vi "Roller IR Logic.vi"(11 "Roller Command In":T2) -> (3 "Roller Command Out":T2, 5 "State":T1)   [LabVIEW 2013]
uses:
  Roller Control.ctl
  Roller Mode.ctl
  Common Code/IR Logic State.ctl
  Common Code/Change Detect Boolean.vi
  Utilities/TimeManager.vi
  Robot Global Data.vi
panel:
  out "IR":cluster{"f":dbl, "f":dbl, "f":dbl}(graph)
  out "Chart":cluster{dbl}(graph)
  in  "Roller/Back IR":bool caption="Back"
  in  "Roller/Center IR":bool caption="Center"
  in  "Roller/Front IR":bool caption="Front"
  in  "To Center Timeout":dbl
  in  "Entry Timeout":dbl
  in  "Verify Center time":dbl
  # "Debugging controls under this box"
  # "IR"
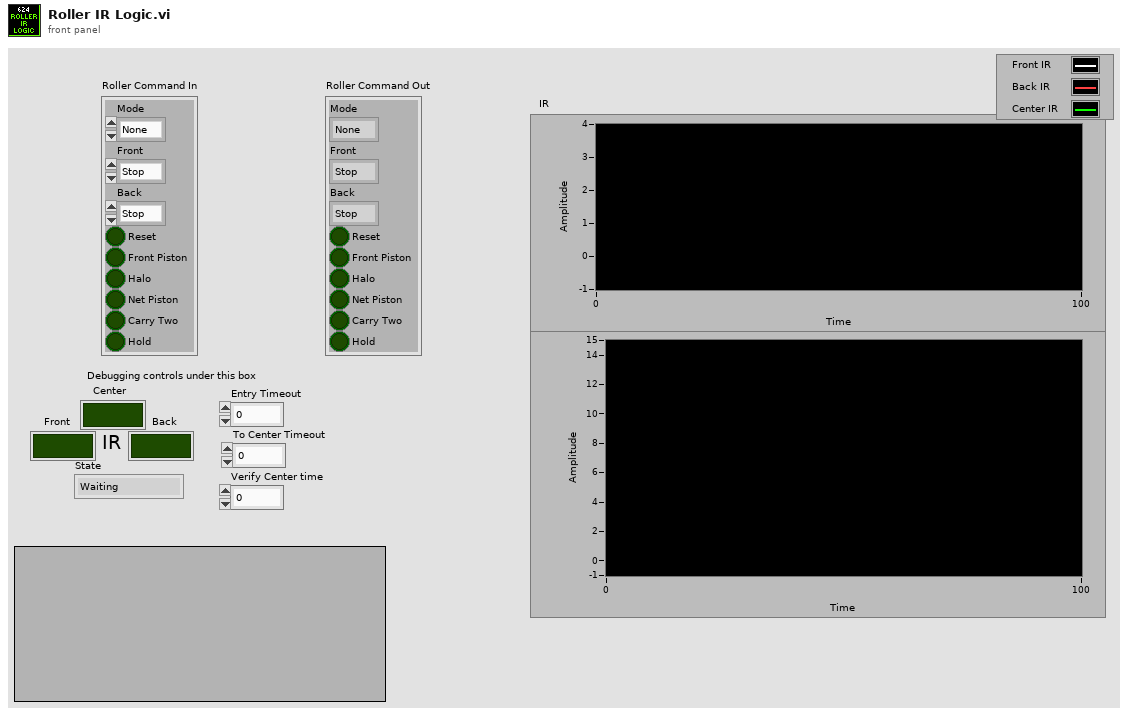
[diagram p1: front panel]
types:
  T1 = typedef "IR Logic State.ctl" = enum16{"Waiting", "Requested", "Loading", "Full", "Wait for Center", "Carry", "Full Carry", "Holding"}
  T2 = typedef "Roller Control.ctl" = cluster{"Mode":T3, "Front":enum16{"Stop", "Forward", "Reverse"}, "Back":enum16{"Stop", "Forward", "Reverse"}, "Reset":bool, "Front Piston":bool, "Halo":bool, "Net Piston":bool, "Carry Two":bool, "Hold":bool}
  T3 = typedef "Roller Mode.ctl" = enum16{"None", "Front", "Back", "Both", "Manual"}
  T4 = typedef "Dashboard UDP Packet.ctl" = cluster{"Camera":T5, "Gyro":T6, "Encoder":T8, "Auto Shift":T9, "Auton":T10, "Drive/Ramp X":dbl, "Drive/Ramp Y":dbl, "Drive/Battery Cutoff":dbl, "Pressure/Compressor Min Voltage":dbl, "Pressure/Compressor Delay":dbl, "Controller/Strafe Correction":bool, "Shooter":T11, "Rollers":T12, "Abort":bool, "Finish":bool, "Shooter Halo Time":dbl, "IR Halo Sustain Time":dbl, "Disable Compressor":bool}
  T5 = typedef "Camera Controls.ctl" = cluster{"Camera/View Angle X":dbl, "Camera/Goal Track Timeout":dbl, "Camera/View Angle Y":dbl, "Camera/Goal Exposure":dbl, "Camera/Vision Receive Timeout":dbl, "Camera/Offset 1":dbl, "Camera/Offset 2":dbl}
  T6 = typedef "Gyro Controls.ctl" = cluster{"Gyro/Angle Tolerance":dbl, "Gyro/Steer Closeness Threshold":dbl, "Steer PID":T7, "Steer Close PID":T7}
  T7 = typedef "PID Params.ctl" = cluster{"max":dbl, "min":dbl, "P":dbl, "I":dbl, "D":dbl}
  T8 = typedef "Encoder Controls.ctl" = cluster{"Encoders/Reset":bool, "Encoders/Omni Constant":dbl, "Encoders/Omni Tick Constant":dbl, "Encoders/Left Constant":dbl, "Encoders/Right Constant":dbl, "Encoders/Right Tick Constant":dbl}
  T9 = typedef "Auto Shift Controls.ctl" = cluster{"AutoShift/Upshift Throttle Accel":dbl, "AutoShift/Speed Threshold":dbl, "AutoShift/Upshift Throttle":dbl, "AutoShift/Upshift Accel":dbl, "AutoShift/Downshift Accel":dbl, "AutoShift/Downshift Throttle":dbl, "AutoShift/Delay":dbl, "AutoShift/Enabled":bool}
  T10 = typedef "Auton Controls.ctl" = cluster{"Auton/Left Shoot X-Coord":dbl, "Auton/Right Shoot X-Coord":dbl, "DistDrive/Distance Stop Threshold":dbl, "DistDrive/Max Stop Speed":dbl, "Auton/Back Piston Time":dbl, "Auton/Manual Hot":bool, "Auton/Manual Hot Right":bool, "Default X PID":T7, "Default Y PID":T7}
  T11 = typedef "Shooter Controls.ctl" = cluster{"Shooter/Reset Time":dbl, "Shooter/Release Delay":dbl, "Shooter/Pressure Steady Time":dbl, "Shooter/Misfire Delay":dbl, "Shooter/Ball Settle Time":dbl, "Shooter/Line IR Delay":dbl, "Pressure/Upper PSI Time":dbl, "Pressure/Lower PSI Time":dbl, "Shooter/Punch Delay":dbl, "Shooter/Target Pressure":dbl, "Pressure/Line B":dbl, "Pressure/Line M":dbl, "Pressure/Shooter M":dbl, "Pressure/Shooter B":dbl}
  T12 = typedef "Roller Controls.ctl" = cluster{"Roller/Load IRs Verify Time":dbl, "Roller/Center IR Latch Time":dbl, "Roller/Speed Front":dbl, "Roller/Speed Back":dbl, "Roller/Entry Timeout":dbl, "Roller/To Center Timeout":dbl, "Roller/Sustain Time":dbl, "Roller/Verify Center Time":dbl}
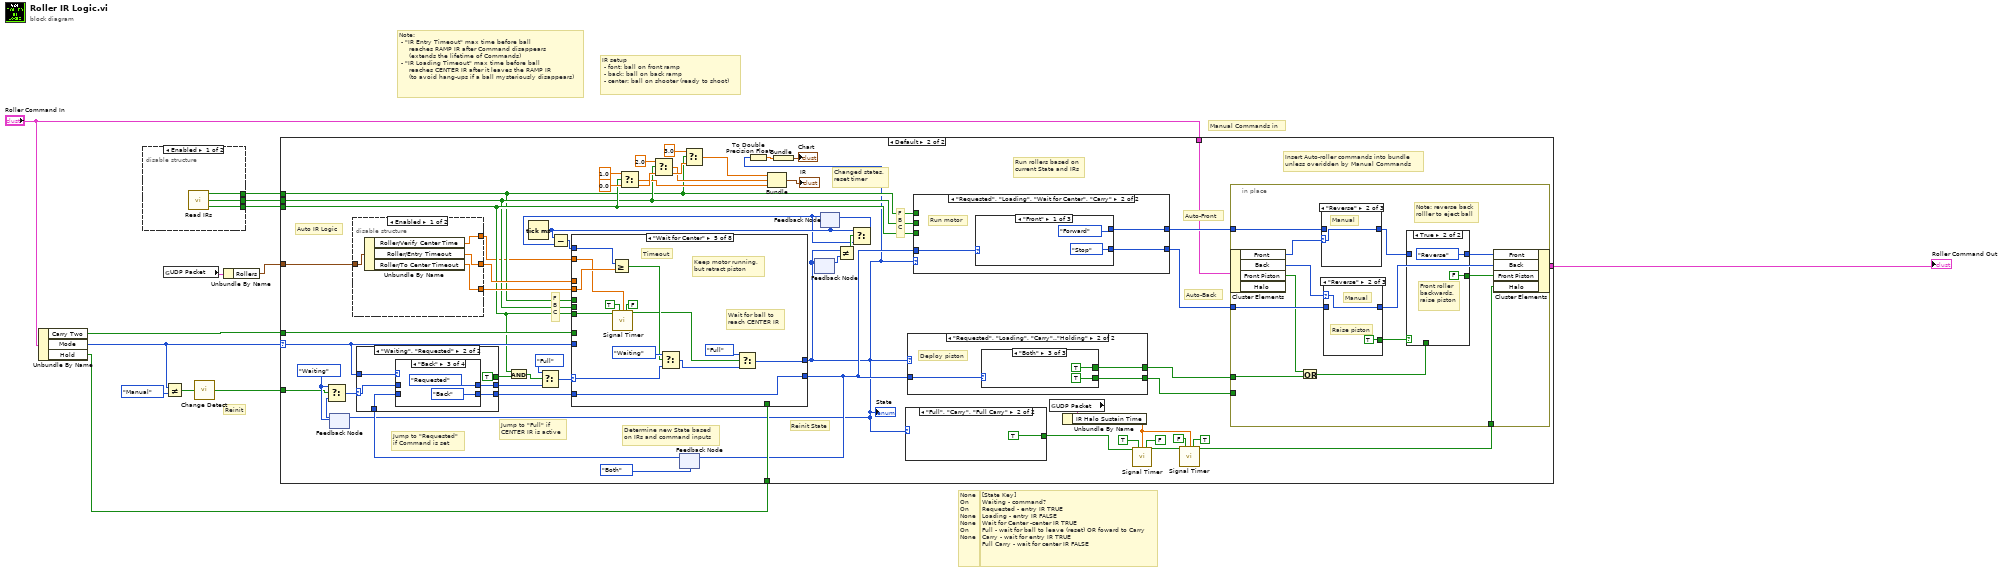
[diagram p0: block diagram]
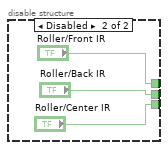
[diagram p2: hidden frame]
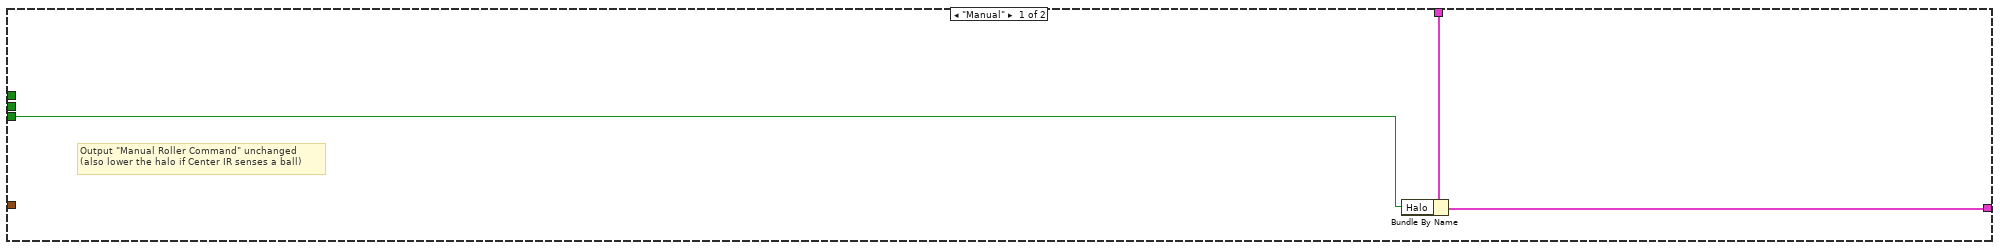
[diagram p3: hidden frame]
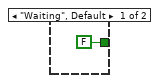
[diagram p4: hidden frame]
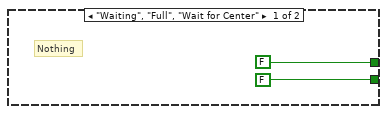
[diagram p5: hidden frame]
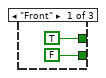
[diagram p6: hidden frame]
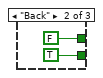
[diagram p7: hidden frame]
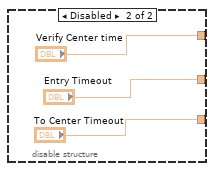
[diagram p13: hidden frame]
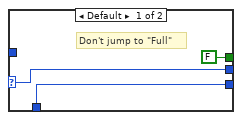
[diagram p14: hidden frame]
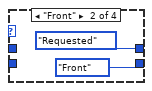
[diagram p16: hidden frame]
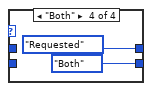
[diagram p17: hidden frame]
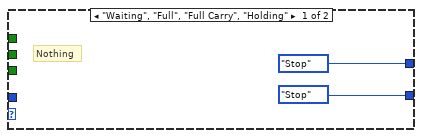
[diagram p18: hidden frame]
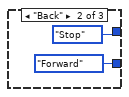
[diagram p19: hidden frame]
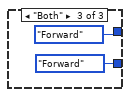
[diagram p20: hidden frame]
diagram:
  # "None\nOn\nOn\nNone\nNone\nOn\nNone"
  # "[State Key]\nWaiting - command?\nRequested - entry IR TRUE\nLoading - entry IR FALSE\nWait for Center -center IR TRUE\nFull - wait for ball to leave (reset) OR foward to Carry\nCarry - wait for entry IR TRUE\nFull Carry - wait for center IR FALSE"
  # "Manual Commands in"
  # "Reinit"
  # "Note:\n - \"IR Entry Timeout\" max time before ball\n     reaches RAMP IR after Command disappears\n     (extends the lifetime of Commands)\n - \"IR Loading Timeout\" max time before ball\n     reaches CENTER IR after it leaves the RAMP IR\n     (to avoid hang-ups if a ball mysteriously disappears)"
  # "IR setup\n - font: ball on front ramp\n - back: ball on back ramp\n - center: ball on shooter (ready to shoot)"
  n1 = Unbundle By Name("Roller Command In") -> ("Carry Two"=w6:bool, "Mode"=w8:T3, "Hold"=w5:bool)
  n2 = disable-structure shown="Enabled" {
    disable-tunnel: [w16 "Roller/Front IR"] -> w13
    disable-tunnel: [w15 "Roller/Back IR"] -> w7
    disable-tunnel: [w14 "Roller/Center IR"] -> w12
    frame Enabled {
      n3 = call "Read IRs.vi"() -> ("Center"=w14:bool, "Back"=w15:bool, "Front"=w16:bool)  [unwired: 2 in, 1 out]
    }
    frame Disabled {
    }
  }
  n4 = global read "Robot Global Data.vi" "UDP Packet"() -> (w3:T4)
  n5 = Not Equal?(x=w8, y=Roller_Mode."Manual" ("x")) -> (x != y?=w4:bool)
  n6 = call-poly "Change Detect.vi"("In"=w4) -> ("Changed?"=w10:bool)
  n7 = Unbundle By Name(w3) -> ("Rollers"=w2:T12)
  n8 = case shown="Default" w8 {
    selector: w8 -> [_ w69]
    tunnel: "Roller Command In" -> [w22 w55]
    tunnel: [w21 w67] -> w1
    tunnel: w10 -> [_ w54]
    tunnel: w13 -> [_ w41]
    tunnel: w7 -> [_ w42]
    tunnel: w12 -> [w20 w43]
    tunnel: w6 -> [_ w58]
    tunnel: w5 -> [_ w56]
    tunnel: w2 -> [_ w33]
    frame "Manual" {
      # "Output \"Manual Roller Command\" unchanged\n(also lower the halo if Center IR senses a ball)"
      n9 = Bundle By Name(cluster=w22, "Halo"=w20) -> (w21:T2)
    }
    frame Default {
      w48 = 0.0 ("f")
      w70 = IR_Logic_State."Waiting"
      # "Reinit State"
      # "Auto-Front"
      # "Auto-Back"
      # "Auto IR Logic"
      # "Changed states,\nreset timer"
      # "Jump to \"Requested\"\nif Command is set"
      # "Jump to \"Full\" if\nCENTER IR is active"
      # "Insert Auto-roller commands into bundle\nunless overidden by Manual Commands"
      # "Run rollers based on\ncurrent State and IRs"
      # "Determine new State based\non IRs and command inputs"
      # "F\nB\nC"
      # "F\nB\nC"
      n10 = feedback #1(w70) -> (w71:T1)
      n11 = Select(t=w70, s=w54, f=w71) -> (s? t:f=w73:T1)
      n12 = disable-structure shown="Enabled" {
        disable-tunnel: [w117 "Entry Timeout"] -> w77
        disable-tunnel: [w116 "To Center Timeout"] -> w76
        disable-tunnel: [w118 "Verify Center time"] -> w37
        disable-tunnel: w33 -> [w115 _]
        frame Enabled {
          n13 = Unbundle By Name(w115) -> ("Roller/Verify Center Time"=w118:dbl, "Roller/Entry Timeout"=w117:dbl, "Roller/To Center Timeout"=w116:dbl)
        }
        frame Disabled {
        }
      }
      n14 = Tick Count (ms)() -> (millisecond timer value=w63:u32)
      n15 = Select(t=1.0, s=w43, f=w48) -> (s? t:f=w44:dbl)
      n16 = Select(t=2.0, s=w42, f=w48) -> (s? t:f=w45:dbl)
      n17 = feedback #2(enum16{"Front", "Back", "Both"}."Both") -> (w39:enum16{"Front", "Back", "Both"})
      n18 = case shown="\"Waiting\", \"Requested\"" w73 {
        selector: w73 -> [w124 w128]
        tunnel: [w124 w130] -> w74
        tunnel: w69 -> [_ w129]
        tunnel: [FALSE TRUE] -> w57
        tunnel: w39 -> [w122 w125]
        tunnel: [w122 w126] -> w38
        frame Default {
          # "Don't jump to \"Full\""
        }
        frame "Waiting", "Requested" {
          n19 = case shown="\"Back\"" w129 {
            tunnel: [w132 IR_Logic_State."Requested" IR_Logic_State."Requested" IR_Logic_State."Requested"] -> w130
            tunnel: w128 -> [w132 _ _ _]
            tunnel: [w131 enum16{"Front", "Back", "Both"}."Front" enum16{"Front", "Back", "Both"}."Back" enum16{"Front", "Back", "Both"}."Both"] -> w126
            tunnel: w125 -> [w131 _ _ _]
            frame "None", Default {
            }
            frame "Front" {
            }
            frame "Back" {
            }
            frame "Both" {
            }
          }
        }
      }
      n20 = And(x=w43, y=w57) -> (x .and. y?=w59:bool)
      n21 = Select(t=IR_Logic_State."Full", s=w59, f=w74) -> (s? t:f=w72:T1)
      n22 = Select(t=3.0, s=w41, f=w48) -> (s? t:f=w46:dbl)
      n23 = Bundle("f"=w46, "f"=w45, "f"=w44) -> (→"IR":cluster{"f":dbl, "f":dbl, "f":dbl})  [unwired: 1 in]
      n24 = feedback #3() -> (w65:T1)  [unwired: 1 in]
      n25 = feedback #4(w63) -> (w61:u32)
      n26 = Subtract(x=w63, y=w61) -> (x-y=w64:u32)
      n27 = case shown="\"Wait for Center\"" w72 {
        selector: w72 -> [w150 w166 w193 w199 w211 w221 w247 w264]
        tunnel: [w150 w167 w187 w202 w215 w226 w246 w263] -> w32
        tunnel: w41 -> [_ w156 w192 _ _ _ w243 _]
        tunnel: w42 -> [_ w154 w189 _ _ _ w242 _]
        tunnel: w43 -> [_ _ _ _ w208 w225 _ w265]
        tunnel: w77 -> [_ w153 _ _ _ _ _ _]
        tunnel: w76 -> [_ _ _ _ w213 _ _ _]
        tunnel: w69 -> [_ w163 _ _ _ w219 _ w261]
        tunnel: w64 -> [_ _ _ _ w214 _ _ _]
        tunnel: w58 -> [_ _ _ _ _ w224 _ _]
        tunnel: w56 -> [_ _ w185 w201 _ _ _ _]
        tunnel: [w151 w152 w184 w198 w203 w222 w241 w262] -> w36
        tunnel: w38 -> [w151 w157 w184 w198 w203 w220 w245 w262]
        tunnel: w37 -> [_ _ _ _ w204 _ _ _]
        frame "Waiting" {
          # "Wait for a Command"
        }
        frame "Requested" {
          # "Entry Timeout"
          # "Wait for ball to reach IR"
          n28 = case shown="\"Both\"" w157 {
            selector: w157 -> [w169 w172 w177]
            tunnel: [Roller_Mode."Front" ("Command 2") Roller_Mode."Back" ("Command 2") Roller_Mode."Both" ("Command 2")] -> w162
            tunnel: w156 -> [w170 _ w178]
            tunnel: [w170 w173 w182] -> w155
            tunnel: w154 -> [_ w173 w179]
            tunnel: [w169 w172 w181] -> w152
            frame "Front" {
            }
            frame "Back" {
            }
            frame "Both" {
              n29 = Or(x=w178, y=w179) -> (x .or. y?=w182:bool)
              n30 = Select(t=enum16{"Front", "Back", "Both"}."Back", s=w179, f=w177) -> (s? t:f=w180:enum16{"Front", "Back", "Both"})
              n31 = Select(t=enum16{"Front", "Back", "Both"}."Front", s=w178, f=w180) -> (s? t:f=w181:enum16{"Front", "Back", "Both"})
            }
          }
          n32 = Select(t=IR_Logic_State."Loading", s=w155, f=w166) -> (s? t:f=w168:T1)
          n33 = Equal?(x=w162, y=w163) -> (x = y?=w159:bool)
          n34 = call "Signal Timer.vi"("Input"=w159, "Edge"=FALSE, "Interval"=w153, "Pull"=TRUE) -> ("Filtered Output"=w158:bool)  [unwired: 11 in]
          n35 = Select(t=w168, s=w158, f=IR_Logic_State."Waiting") -> (s? t:f=w167:T1)
        }
        frame "Loading" {
          # "Reset rollers to \"Hold\" ball"
          # "Wait for ball to\nleave IR"
          n36 = case shown="\"Front\"" w184 {
            tunnel: w192 -> [w195 _ _]
            tunnel: [w195 w196 FALSE ("Back")] -> w190
            tunnel: w189 -> [_ w196 _]
            frame "Front" {
            }
            frame "Back" {
            }
            frame Default {
              # "bad state\n[exit]"
            }
          }
          n37 = Not(x=w190) -> (.not. x?=w191:bool)
          n38 = Select(t=IR_Logic_State."Wait for Center", s=w191, f=w193) -> (s? t:f=w188:T1)
          n39 = Select(t=IR_Logic_State."Holding", s=w185, f=w188) -> (s? t:f=w187:T1)
        }
        frame "Holding" {
          # "(stop motor, but keep piston down)"
          # "Back to Loading\nwhen done Holding"
          n40 = Select(t=w199, s=w201, f=IR_Logic_State."Loading") -> (s? t:f=w202:T1)
        }
        frame "Wait for Center" {
          # "Keep motor running,\nbut retract piston"
          # "Timeout"
          # "Wait for ball to\nreach CENTER IR"
          n41 = Greater Or Equal?(x=w214, y=w213) -> (x >= y?=w209:bool)
          n42 = call "Signal Timer.vi"("Input"=w208, "Edge"=TRUE, "Interval"=w204, "Pull"=FALSE) -> ("Filtered Output"=w207:bool)  [unwired: 11 in]
          n43 = Select(t=IR_Logic_State."Waiting", s=w209, f=w211) -> (s? t:f=w210:T1)
          n44 = Select(t=IR_Logic_State."Full", s=w207, f=w210) -> (s? t:f=w215:T1)
        }
        frame "Full" {
          n45 = case shown="\"Front\"" w219 {
            tunnel: [enum16{"Front", "Back", "Both"}."Front" enum16{"Front", "Back", "Both"}."Back" enum16{"Front", "Back", "Both"}."Both" _] -> w217
            tunnel: [TRUE TRUE TRUE FALSE] -> w218
            frame "Front" {
            }
            frame "Back" {
            }
            frame "Both" {
            }
            frame Default {
            }
          }
          n46 = And(x=w218, y=w224) -> (x .and. y?=w223:bool)
          n47 = case shown="True" w223 {
            tunnel: [w236 IR_Logic_State."Carry"] -> w226
            tunnel: w225 -> [w237 _]
            tunnel: [w234 w239] -> w222
            tunnel: w221 -> [w235 _]
            tunnel: w220 -> [w234 _]
            tunnel: w217 -> [_ w239]
            frame False {
              # "Wait until ball disappears\nfrom CENTER IR (ex: after shooting)"
              n48 = Select(t=w235, s=w237, f=IR_Logic_State."Waiting") -> (s? t:f=w236:T1)
            }
            frame True {
              # "Continue to \"Carry\" case"
            }
          }
        }
        frame "Carry" {
          # "(similar to Requested)"
          # "Note: direction comes from \"Full\" (from command)"
          # "Wait for ball to reach IR"
          n49 = case shown="\"Both\"" w245 {
            selector: w245 -> [w249 w251 w255]
            tunnel: [w250 w252 w254] -> w244
            tunnel: w243 -> [w250 _ w257]
            tunnel: w242 -> [_ w252 w258]
            tunnel: [w249 w251 w256] -> w241
            frame "Front" {
            }
            frame "Back" {
            }
            frame "Both" {
              n50 = Or(x=w257, y=w258) -> (x .or. y?=w254:bool)
              n51 = Select(t=enum16{"Front", "Back", "Both"}."Back", s=w258, f=w255) -> (s? t:f=w260:enum16{"Front", "Back", "Both"})
              n52 = Select(t=enum16{"Front", "Back", "Both"}."Front", s=w257, f=w260) -> (s? t:f=w256:enum16{"Front", "Back", "Both"})
            }
          }
          n53 = Select(t=IR_Logic_State."Full Carry", s=w244, f=w247) -> (s? t:f=w246:T1)
        }
        frame "Full Carry" {
          n54 = case shown="False" w265 {
            tunnel: w264 -> [w266 w271]
            tunnel: [w268 w271] -> w263
            tunnel: w261 -> [w267 _]
            frame False {
              # "Return to Load when center IR\nreads FALSE"
              n55 = case shown="\"None\", Default" w267 {
                tunnel: [w269 IR_Logic_State."Loading"] -> w268
                tunnel: w266 -> [w269 _]
                frame "None", Default {
                  # "Wait in this case"
                }
                frame "Front".."Both" {
                }
              }
            }
            frame True {
              # "Wait for ball to\nleave center IR"
            }
          }
        }
      }
      "State" <- w32
      n56 = feedback-in #1(w32) -> ()
      n57 = feedback-in #2(w36) -> ()
      n58 = To Double Precision Float(number=w32) -> (double precision float=w52:dbl)
      n59 = Bundle(w52) -> (→"Chart":cluster{dbl})  [unwired: 1 in]
      n60 = feedback-in #3(w32) -> ()
      n61 = Not Equal?(x=w32, y=w65) -> (x != y?=w62:bool)
      n62 = Select(t=w63, s=w62, f=w61) -> (s? t:f=w60:u32)
      n63 = feedback-in #4(w60) -> ()
      n64 = case shown="\"Full\", \"Carry\", \"Full Carry\"" w32 {
        tunnel: [FALSE TRUE] -> w31
        frame "Waiting", Default {
        }
        frame "Full", "Carry", "Full Carry" {
        }
      }
      n65 = case shown="\"Requested\", \"Loading\", \"Carry\"..\"Holding\"" w32 {
        tunnel: [FALSE w84] -> w35
        tunnel: [FALSE w83] -> w34
        tunnel: w36 -> [_ w82]
        frame "Waiting", "Full", "Wait for Center" {
          # "Nothing"
        }
        frame "Requested", "Loading", "Carry".."Holding" {
          # "Deploy piston"
          n66 = case shown="\"Both\"" w82 {
            tunnel: [TRUE FALSE TRUE] -> w84
            tunnel: [FALSE TRUE TRUE] -> w83
            frame "Front" {
            }
            frame "Back" {
            }
            frame "Both" {
            }
          }
        }
      }
      n67 = case shown="\"Requested\", \"Loading\", \"Wait for Center\", \"Carry\"" w32 {
        tunnel: [enum16{"Stop", "Forward", "Reverse"}."Stop" ("Front") w142] -> w68
        tunnel: [enum16{"Stop", "Forward", "Reverse"}."Stop" ("Front") w141] -> w66
        tunnel: w43 -> [_ _]
        tunnel: w42 -> [_ _]
        tunnel: w41 -> [_ _]
        tunnel: w36 -> [_ w143]
        frame "Waiting", "Full", "Full Carry", "Holding" {
          # "Nothing"
        }
        frame "Requested", "Loading", "Wait for Center", "Carry" {
          # "Run motor"
          n68 = case shown="\"Front\"" w143 {
            tunnel: [enum16{"Stop", "Forward", "Reverse"}."Forward" ("Front") enum16{"Stop", "Forward", "Reverse"}."Stop" ("Front") enum16{"Stop", "Forward", "Reverse"}."Forward" ("Front")] -> w142
            tunnel: [enum16{"Stop", "Forward", "Reverse"}."Stop" ("Front") enum16{"Stop", "Forward", "Reverse"}."Forward" ("Front") enum16{"Stop", "Forward", "Reverse"}."Forward" ("Front")] -> w141
            frame "Front" {
            }
            frame "Back" {
            }
            frame "Both" {
            }
          }
        }
      }
      n69 = global read "Robot Global Data.vi" "UDP Packet"() -> (w28:T4)
      n70 = Unbundle By Name(w28) -> ("IR Halo Sustain Time"=w24:dbl)
      n71 = call "Signal Timer.vi"("Input"=w31, "Edge"=TRUE, "Interval"=w24, "Pull"=FALSE) -> ("Filtered Output"=w27:bool)  [unwired: 11 in]
      n72 = call "Signal Timer.vi"("Input"=w27, "Edge"=FALSE, "Interval"=w24, "Pull"=TRUE) -> ("Filtered Output"=w23:bool)  [unwired: 11 in]
      n73 = in-place {
        in-place-border: w68 -> [w100]
        in-place-border: w66 -> [w99]
        in-place-border: w35 -> [w97]
        in-place-border: w34 -> [_]
        in-place-border: w23 -> [w96]
        # "Note: reverse back\nrolller to eject ball"
        n74 = in-place-cluster #5(w55) -> ("Front"=w103:enum16{"Stop", "Forward", "Reverse"}, "Back"=w102:enum16{"Stop", "Forward", "Reverse"}, "Front Piston"=w98:bool)  [unwired: 1 out]
        n75 = Or(x=w98, y=w97) -> (x .or. y?=w92:bool)
        n76 = case shown="\"Reverse\"" w103 {
          selector: w103 -> [w112 w113 _]
          tunnel: [w112 w113 w114] -> w94
          tunnel: w100 -> [_ _ w114]
          frame Default {
            # "Manual"
          }
          frame "Reverse" {
            # "Manual"
          }
          frame "Stop" {
            # "Auto allowed"
          }
        }
        n77 = case shown="\"Reverse\"" w102 {
          selector: w102 -> [w108 w110 _]
          tunnel: [w108 w110 w111] -> w101
          tunnel: w99 -> [_ _ w111]
          tunnel: [_ TRUE ("x") _] -> w95
          frame Default {
            # "Manual"
          }
          frame "Reverse" {
            # "Raise piston"
            # "Manual"
          }
          frame "Stop" {
            # "Auto allowed"
          }
        }
        n78 = case shown="True" w95 {
          tunnel: w94 -> [w105 _]
          tunnel: [w105 enum16{"Stop", "Forward", "Reverse"}."Reverse" ("Front")] -> w93
          tunnel: w92 -> [w104 _]
          tunnel: [w104 FALSE] -> w91
          frame False {
          }
          frame True {
            # "Front roller\nbackwards,\nraise piston"
          }
        }
        n79 = in-place-cluster #5("Front"=w93, "Back"=w101, "Front Piston"=w91, "Halo"=w96) -> (w67:T2)
      }
    }
  }
  "Roller Command Out" <- w1
